vi "FPGA_SPI_interface.vi"(8 "Frames to Write":u8[](array[numeric]), 10 "error in":errorcluster, 11 "FPGA VI Reference In":T1) -> (0 "Frames Read":u8[](array[numeric]), 2 "error out":errorcluster, 3 "FPGA VI Reference Out":T1)   [LabVIEW 2016]
uses:
  FPGA Bitfiles/FPGA_defref.ctl
  <vilib>/Utility/error.llb/Error Cluster From Error Code.vi
  <vilib>/rvi/errors/niLvFpgaAdjustHostInterfaceError.vi
  <vilib>/rvi/interface/nirviMethod/nirviMethod.xnode
  FPGA Bitfiles/nRF24Communicati_FPGATarget_FPGATest_lnf7SjQfCOM.lvbitx
  FPGATest.vi
  <vilib>/rvi/interface/nirviReadWriteControl/nirviReadWriteControl.xnode
  NiFpgaLv.dll
  <vilib>/rvi/errors/niLvFpgaMergeErrorWithErrorCode.vi
  <vilib>/FPGAPlugInAG/roboRIO/niLvFpga_ReadFifo_roboRIO.vi
  <vilib>/FPGAPlugInAG/roboRIO/niLvFpga_WriteFifo_roboRIO.vi
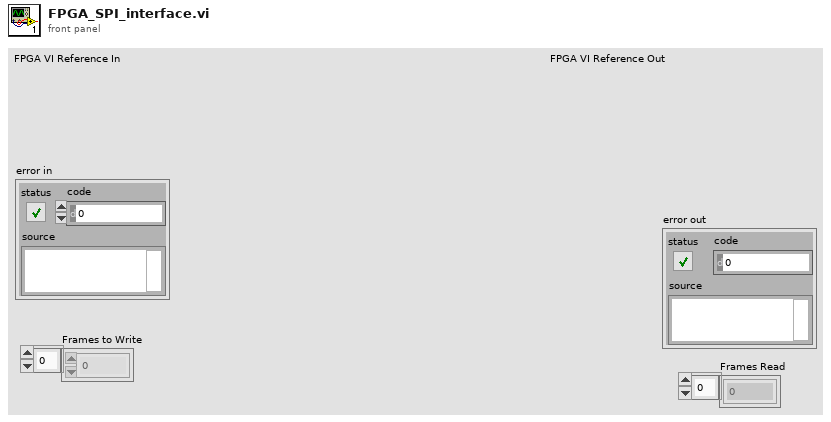
[diagram p1: front panel]
types:
  T1 = typedef "FPGA_defref.ctl" = refnum<k20>
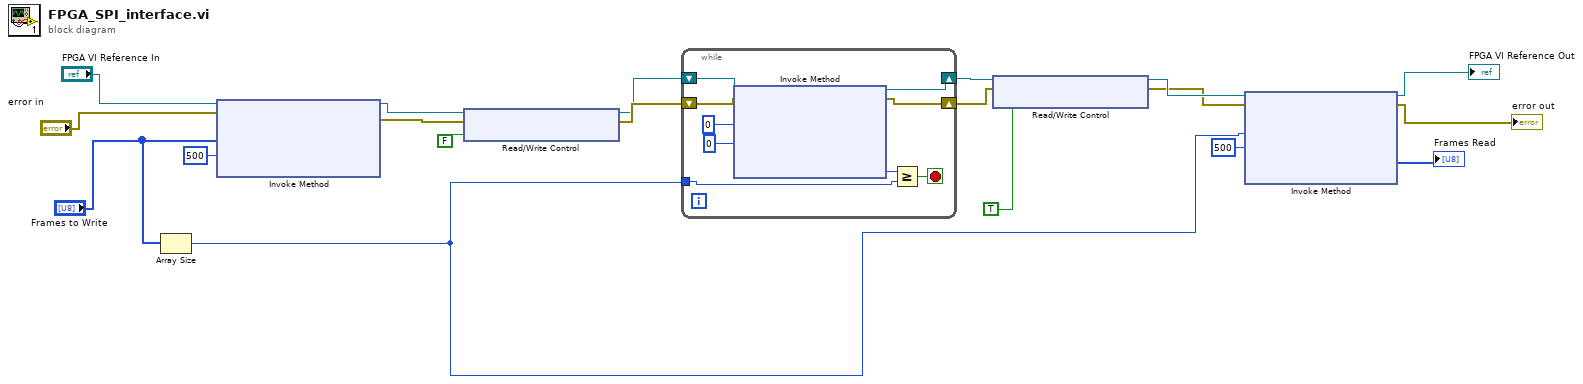
[diagram p0: block diagram]
diagram:
  n1 = Array Size(array="Frames to Write") -> (size(s)=w1:i32)
  n2 = xnode "Invoke Method"("FPGA VI Reference In"="FPGA VI Reference In", "error in"="error in", "Data"="Frames to Write", "Timeout (ms)"=500) -> ("FPGA VI Reference Out"=w15:T1, "error out"=w14:errorcluster)  [unwired: 1 out]
  n3 = xnode "Read/Write Control"("FPGA VI Reference In"=w15, "error in"=w14, "CS"=FALSE) -> ("FPGA VI Reference Out"=w4:T1, "error out"=w5:errorcluster)
  n4 = while {
    shift-right: [w26] -> w3
    shift-left: w5 -> [w28]
    shift-right: [w25] -> w2
    shift-left: w4 -> [w27]
    tunnel: w1 -> [w21]
    stop <- w22 stop-if-true
    n5 = xnode "Invoke Method"("FPGA VI Reference In"=w27, "error in"=w28, "Number of Elements"=u32 0, "Timeout (ms)"=0) -> ("FPGA VI Reference Out"=w25:T1, "error out"=w26:errorcluster, "Elements Remaining"=w20:u32)  [unwired: 1 out]
    n6 = Greater Or Equal?(x=w20, y=w21) -> (x >= y?=w22:bool)
  }
  n7 = xnode "Read/Write Control"("FPGA VI Reference In"=w2, "error in"=w3, "CS"=TRUE) -> ("FPGA VI Reference Out"=w13:T1, "error out"=w12:errorcluster)
  n8 = xnode "Invoke Method"("FPGA VI Reference In"=w13, "error in"=w12, "Number of Elements"=w1, "Timeout (ms)"=500) -> ("FPGA VI Reference Out"=→"FPGA VI Reference Out":T1, "error out"=→"error out":errorcluster, "Data"=→"Frames Read":u8[])  [unwired: 1 out]
